vi "ADS Custom Personality FPGA FPGA.vi"() -> ()   [LabVIEW 2015]
uses:
  FPGA Function.ctl
  <vilib>/LabVIEW Targets/FPGA/cRIO/shared/nicrio_ModuleControls/nicrio_cRIO-9237_DataRatesRing.ctl
  <vilib>/LabVIEW Targets/FPGA/cRIO/shared/nicrio_ModuleControls/nicrio_cRIO-9237_ExcitationVoltageRing.ctl
  <vilib>/Platform/TimedLoop/XDataNode/timing_clust.ctl
  <vilib>/Platform/TimedLoop/XDataNode/nitl_modes.ctl
  <vilib>/Platform/TimedLoop/XDataNode/wakeup.ctl
  <vilib>/LabVIEW Targets/FPGA/cRIO/shared/nicrio_ModuleControls/nicrio_cRIO-9871_BaudRatePrescalerEnum.ctl
  <vilib>/LabVIEW Targets/FPGA/cRIO/shared/nicrio_ModuleControls/nicrio_cRIO-9871_XcvrModeEnum.ctl
  <vilib>/rvi/Emulation/niFpgaGetClockAttributes.vi
  <vilib>/rvi/Emulation/niFpgaSctlEmulationGetInTimedLoop.vi
  <vilib>/rvi/Emulation/niFpgaEmulationReportErrorSimple.vi
  <vilib>/rvi/Emulation/niFpgaCriticalErrorInLSC.vi
  <vilib>/rvi/eio/common/nirviEmuTemplateMethod_errors.vi
  <vilib>/rvi/eio/common/nirviEmuTemplatePropertySet_noerrors.vi
  <vilib>/rvi/Emulation/niFpgaProcessEmulError.vi
  <vilib>/rvi/DataTransferAndStorage/Container/Common/niFpgaContainerGetUniqueNameForEmu.vi
  <vilib>/rvi/DataTransferAndStorage/Container/Common/niFpgaContainerSetEmuInfo.vi
  <vilib>/rvi/eio/common/nirviEmuReportErrorAndStop.vi
  <vilib>/rvi/DataTransferAndStorage/Container/Common/niFpgaContainerExecOnDevCompGetState.vi
  <vilib>/rvi/Emulation/niFpgaEmulationIsFPGAContextNoSignature.vi
  <vilib>/rvi/errors/niFpgaSetErrorForExecOnDevCompSimple.vi
  <vilib>/rvi/FIFO/Fifo_Resource/nirvififoEmulationSetSize.vi
  <vilib>/rvi/FIFO/Fifo_Resource/nirviFifoEmulationQueueMgr.vi
  <instcachedir>/0/nirviFifoEmulationQueueMgr_E5CAEC123FF24DC58D834DCA3CDAA9B5.lvgen/nirviFifoEmulationQueueMgr_E5CAEC123FF24DC58D834DCA3CDAA9B5_001.vi
  <vilib>/rvi/FIFO/Fifo_Resource/nirvififoEmulationDetermineInputValidOut.vi
  <vilib>/rvi/FIFO/Fifo_Resource/nirvififoEmulationCreateLock.vi
  <vilib>/rvi/FIFO/Fifo_Resource/nirvififoEmulationObtainLock.vi
  <vilib>/rvi/FIFO/Fifo_Resource/nirvififoEmulationReleaseLock.vi
  <vilib>/rvi/occurrence/nirviWaitOnOccurrenceBase.vi
  <vilib>/rvi/errors/nirviReportUnexpectedCaseInternalError.vi
  <vilib>/rvi/errors/nirviReportUnexpectedCaseInternalError (U32).vi
  <vilib>/Utility/error.llb/Clear Errors.vi
  <vilib>/rvi/interface/RandomDataEmulation/niFpgaRandomDataHandleErrors.vi
  <vilib>/Platform/TimedLoop/XDataNode/XDataNode.xnode
  <vilib>/eio/EIONode/EIONode.xnode
  <vilib>/eio/EIOPropertyNode/EIOPropertyNode.xnode
  <vilib>/rvi/LocalResourceManager/LocalResourceManager.xnode
  <vilib>/rvi/DataTransferAndStorage/Container/XNode/niFpgaContainer.xnode
  <vilib>/rvi/FIFO/Fifo_Resource/niFpgaFifoEmulationRefIn.vi
  <vilib>/eio/EIOMethodNode/EIOMethodNode.xnode
  <vilib>/Platform/TimedLoop/XDataNode/XDNodeRunTimeDep.lvlib
  <vilib>/NI Veristand/FPGA/NI_VS FPGA Support.lvlib
  <userlib>/_NI VeriStand FPGA Support/NI VeriStand FPGA Clock Support/NI_VS FPGA Clock Support.lvlib
  <vilib>/rvi/eio/common/nirviEmuTemplatePropertyGet_errors.vi
  <vilib>/rvi/eio/common/nirviEmuTemplatePropertyGet_noerrors.vi
  <vilib>/rvi/eio/common/nirviEmuTemplatePropertySet_errors.vi
panel:
  out "Count 6":u32
  out "Count 5":u32
  out "Count 4":u32
  out "Count 3":u32
  out "Count 2":u32
  in  "Edge":enum8{"Either", "Rising Edge", "Falling Edge"}(ring)=enum."Rising Edge"
  in  "Reset":bool
  in  "Count Direction":enum16{"Count Down", "Count Up"}(ring)=enum."Count Up"
  out "Count":u32
  in  "Excitation Voltage":T1=2 items=["2.5 Volts", "3.3 Volts", "5.0 Volts", "10.0 Volts", "External Excitation"]
  in  "RecDelay":u32=550
  out "PosComm":fxp<+/-,24,16>[](array[numeric])=[68.78125, 0.0, 0.0, 0.0, 0.0, 0.0]
  in  "Baudrate":u8=4
  in  "SetBaudrate":bool
  out "Time":u32=1
  in  "Baud Rate Divider":u16=9
  in  "9237 Data Rate":T2=1 items=["50.000 kS/s (NI 9237)"=1, "25.000 kS/s (NI 9237)"=2, "16.667 kS/s (NI 9237)"=3, "12.500 kS/s (NI 9237)"=4, "10.000 kS/s (NI 9237)"=5, "8.333 kS/s (NI 9237)"=6, "7.143 kS/s (NI 9237)"=7, "6.250 kS/s (NI 9237)"=8, "5.556 kS/s (NI 9237)"=9, "5.000 kS/s (NI 9237)"=10, "4.545 kS/s (NI 9237)"=11, "4.167 kS/s (NI 9237)"=12, "3.846 kS/s (NI 9237)"=13, "3.571 kS/s (NI 9237)"=14, "3.333 kS/s (NI 9237)"=15, "3.125 kS/s (NI 9237)"=16, "2.941 kS/s (NI 9237)"=17, "2.778 kS/s (NI 9237)"=18, "2.632 kS/s (NI 9237)"=19, "2.500 kS/s (NI 9237)"=20, "2.381 kS/s (NI 9237)"=21, "2.273 kS/s (NI 9237)"=22, "2.174 kS/s (NI 9237)"=23, "2.083 kS/s (NI 9237)"=24, "2.000 kS/s (NI 9237)"=25, "1.923 kS/s (NI 9237)"=26, "1.852 kS/s (NI 9237)"=27, "1.786 kS/s (NI 9237)"=28, "1.724 kS/s (NI 9237)"=29, "1.667 kS/s (NI 9237)"=30, "1.613 kS/s (NI 9237)"=31]
  in  "NoB2Read":i32=48
  in  "ScaleDeg":fxp<+/-,25,16>=2.849609375
  out "ReadData":u8[](array[numeric])=[255, 255, 1, 4, 0, 196, 0, 54, 255, 255, 2, 4, 0, 0, 0, 249, 255, 255, 3, 4, 0, 0, 0, 248, 255, 255, 4, 4, 0, 0, 0, 247, 255, 255, 5, 4, 0, 0, 0, 246, 255, 255, 6, 4, 0, 0, 0, 245, 0, 0, 0, 0, 0, 0, 0, 0] format="%x"
  out "NoC":i32=49
  out "Number of Elements to Read Output":u32=26
  out "PresentPos":u64[](array[numeric])=[688, 0, 0, 210453397552]
  out "WriteData":u8[](array[numeric])=[255, 255, 254, 21, 146, 0, 2, 1, 36, 2, 2, 36, 2, 3, 36, 2, 4, 36, 2, 5, 36, 2, 6, 36, 97, 0, 0, 0, 0, 0]
  out "error out":errorcluster
  in  "SerialFunction":T3=enum."Read"
  in  "PosVal":fxp<+/-,24,16>
  in  "EOS Enabled":bool
  in  "EOS":u8
  out "Timed Out Read":bool
  out "EOS?":bool
  out "Timed Out Write":bool
  in  "_PWM Pulses 0-7":u64[](array[numeric])=[4294967395000, 100000, 100000, 100000, 100000, 100000, 100000, 100000]
  in  "Generate IRQ":bool=TRUE
  in  "Use External Timing":bool
  in  "Write to  RTSI":bool=TRUE
  in  "Loop Rate (usec)":u32=10000
  in  "Start":bool
  # "PWM"
  # "Configuration"
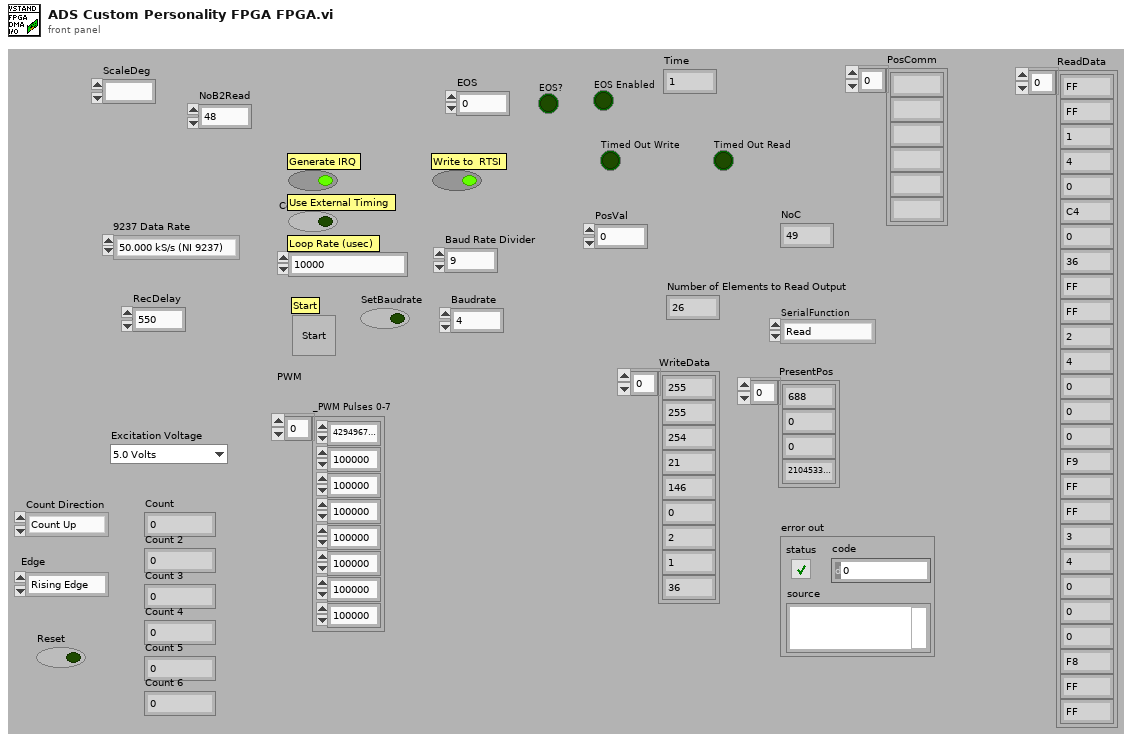
[diagram p1: front panel]
types:
  T1 = typedef "nicrio_cRIO-9237_ExcitationVoltageRing.ctl" = u8
  T2 = typedef "nicrio_cRIO-9237_DataRatesRing.ctl" = u8
  T3 = typedef "FPGA Function.ctl" = enum16{"Do Nothing", "Write", "Read"}
  T4 = typedef "XDNodeRunTimeDep.lvlib/timing_clust.ctl" = cluster{"Expected End [f-1]":u64, "Actual End [f-1]":u64, "Finished Late? [f-1]":bool, "Expected End [i-1]":u64, "Actual End [i-1]":u64, "Finished Late? [i-1]":bool, "Expected Start [i]":u64, "Actual Start [i]":u64, "Expected Start [f]":u64, "Actual Start [f]":u64, "Source Name":string, "Structure Name":string, "Period":i64, "Deadline":i64, "Offset":i64, "Start":i64, "Priority":i32, "Timeout":i32, "Mode":T5, "Wakeup Reason":T6, "Error":errorcluster, "Source Type":string, "Secondary Source Type":string, "Global End Time":u64, "Global Start Time":u64, "Frame Duration":u64, "Iteration Duration":u64, "Assigned CPU":i32, "I/O Scan Engine Mode":u32}
  T5 = typedef "XDNodeRunTimeDep.lvlib/nitl_modes.ctl" = enum32{"No Change", "Process missed periods, maintain original phase", "Discard missed periods, maintain original phase", "Process missed periods, ignore original phase", "Discard missed periods, ignore original phase"}
  T6 = typedef "XDNodeRunTimeDep.lvlib/wakeup.ctl" = enum32{"Normal", "Aborted", "Asynchronous wakeup", "Timing source error", "Timed loop error", "Timeout"}
  T7 = cluster{"9235/9236/9237 AI0":refnum<k21>, "9235/9236/9237 AI1":refnum<k21>, "9235/9236/9237 AI2":refnum<k21>, "9235/9236/9237 AI3":refnum<k21>}
  T8 = cluster{"9215 AI0":refnum<k21>, "9215 AI1":refnum<k21>, "9215 AI2":refnum<k21>, "9215 AI3":refnum<k21>}
  T9 = typedef "nicrio_cRIO-9871_XcvrModeEnum.ctl" = enum8{"4 Wire", "2 Wire DTR Controlled with Echo", "2 Wire DTR Controlled", "2 Wire Auto"}
  T10 = typedef "nicrio_cRIO-9871_BaudRatePrescalerEnum.ctl" = enum8{"1", "4"}
  T11 = cluster{"DO0":refnum<k21>, "DO1":refnum<k21>, "DO2":refnum<k21>, "DO3":refnum<k21>}
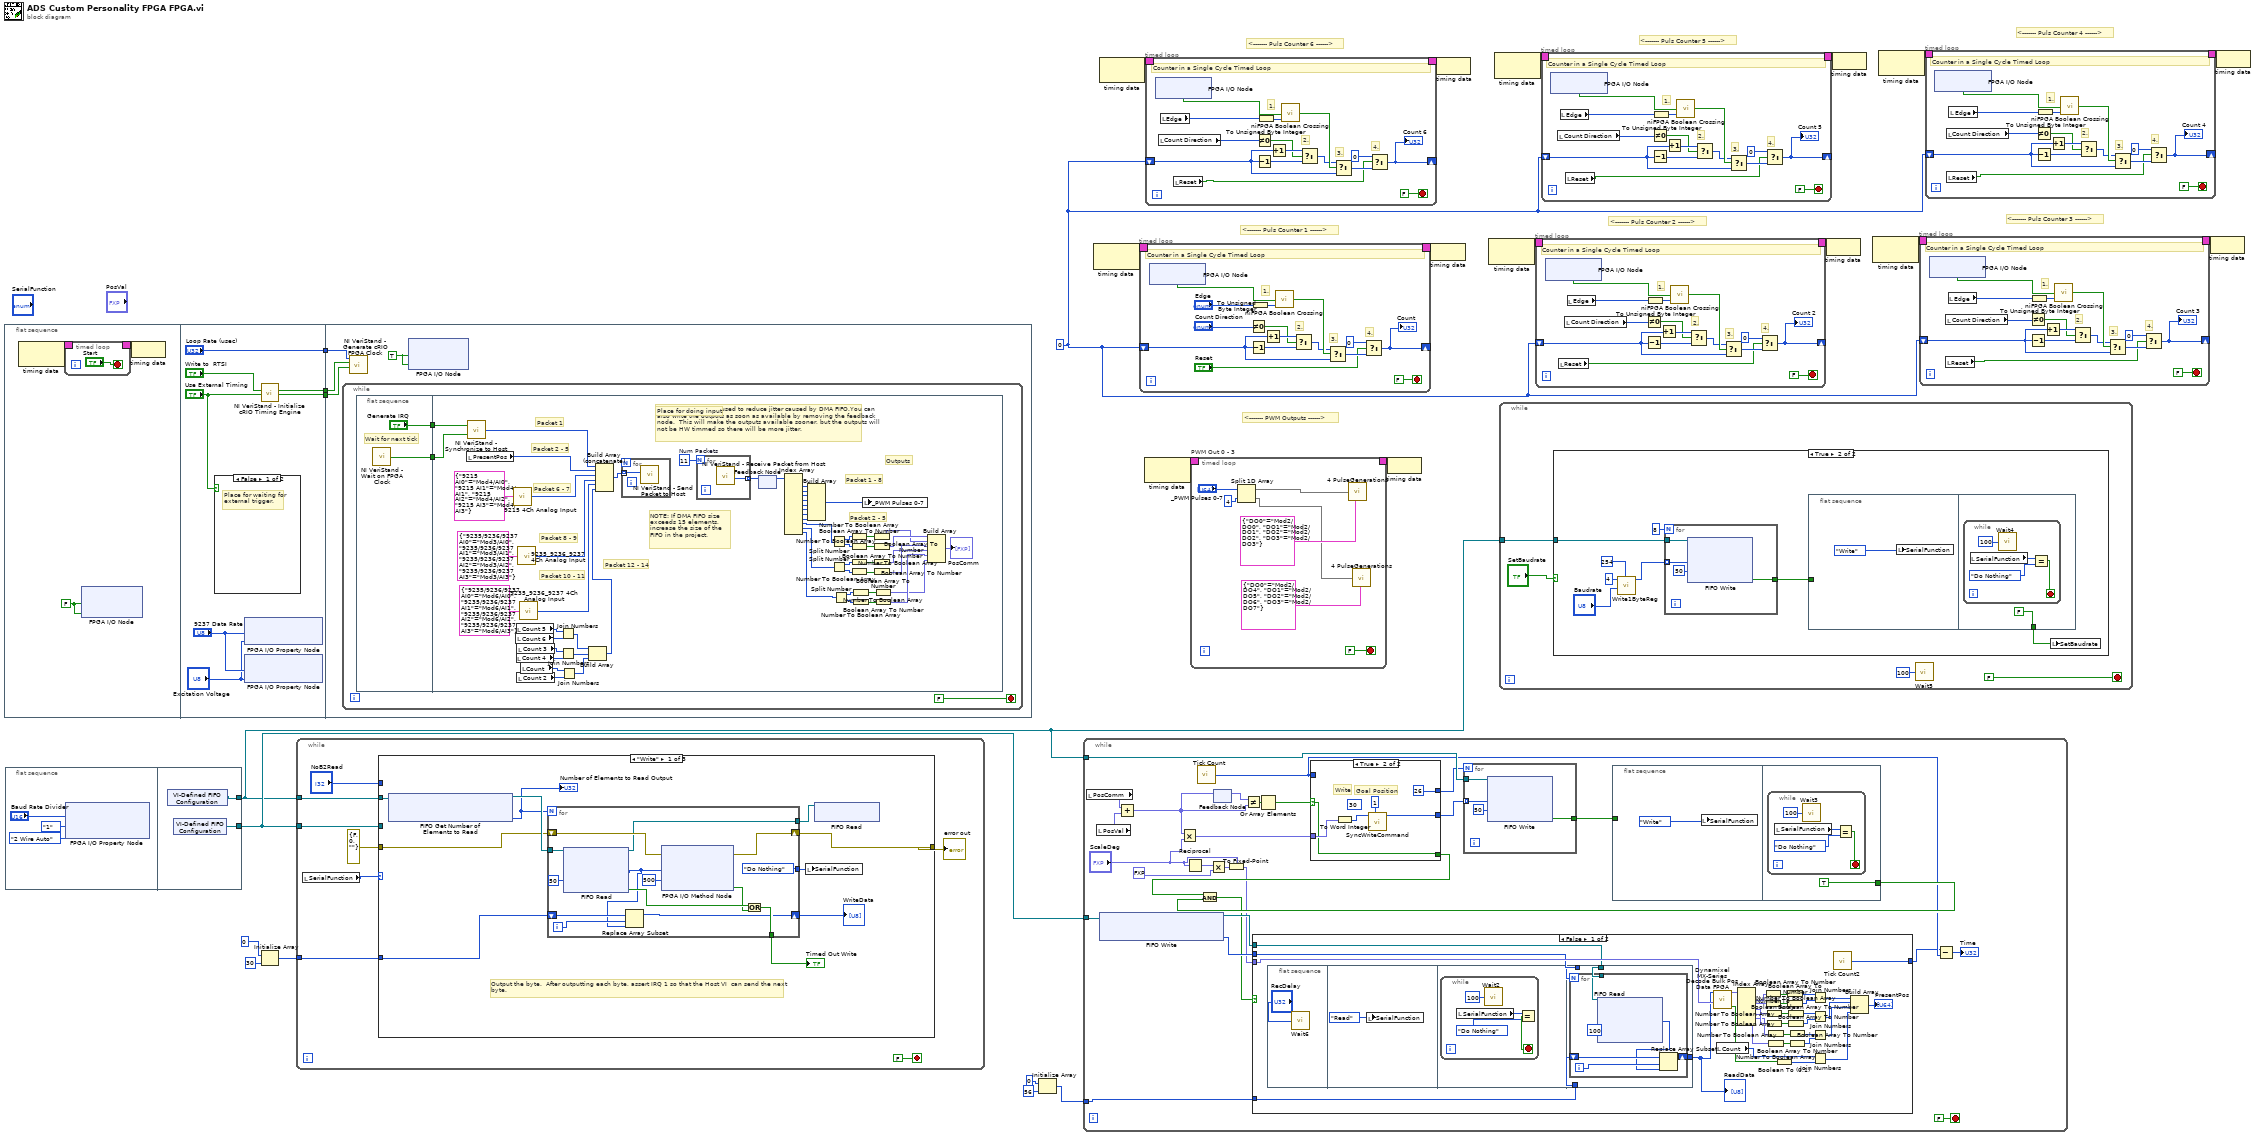
[diagram p0: block diagram]
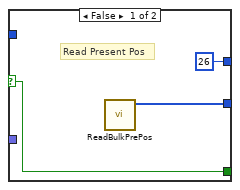
[diagram p4: hidden frame]
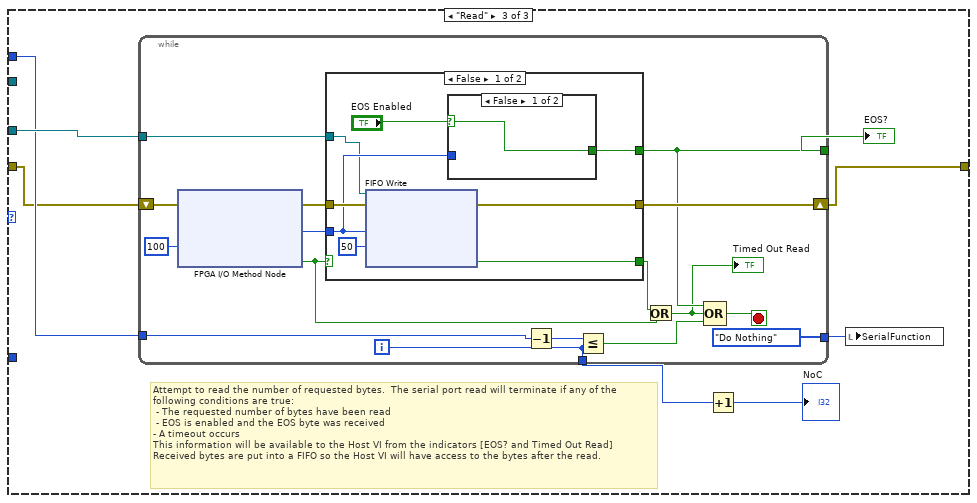
[diagram p6: hidden frame]
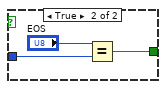
[diagram p7: hidden frame]
diagram:
  w1 = u32 0
  # "<------- Puls Counter 5 ------>"
  # "<------- Puls Counter 4 ------>"
  # "<------- Puls Counter 3 ------>"
  # "<------- Puls Counter 2 ------>"
  # "<------- Puls Counter 6 ------>"
  # "<------- Puls Counter 1 ------>"
  # "<------- PWM Outputs ------>"
  n1 = flat-sequence {
    tunnel: [w38] -> w26
    tunnel: ["Loop Rate (usec)"] -> w25
    tunnel: [w37] -> w22
    tunnel: w26 -> [w45]
    tunnel: w25 -> [w44]
    tunnel: w22 -> [w43]
    frame #0 {
      w27 = FALSE
      n2 = node-c288() -> (w29:T4)  [unwired: 1 out]
      n3 = timed-loop {
        timing: w29 -> [_]
        timing-out: [_] -> w28
        stop <- "Start" stop-if-true
      }
      n4 = xnode "FPGA I/O Node"("Mod3/Start"=w27, "Mod6/Start"=w27) -> ()  [unwired: 2 in, 2 out]
      n5 = node-c288(w28) -> ()
    }
    frame #1 {
      n6 = case shown="False" "Use External Timing" {
        frame False {
          # "Place for waiting for external trigger."
        }
        frame True {
          # "Do not wait on trigger when externally timed."
        }
      }
      n7 = xnode "FPGA I/O Property Node"("Data Rate"="9237 Data Rate", "Excitation Voltage"="Excitation Voltage") -> ()  [unwired: 1 in, 1 out]
      n8 = xnode "FPGA I/O Property Node"("Data Rate"="9237 Data Rate", "Excitation Voltage"="Excitation Voltage") -> ()  [unwired: 1 in, 1 out]
      n9 = call <userlib>:"NI VeriStand - Initialize cRIO Timing Engine.vi"("Use External Timing In"="Use External Timing", "Write to  RTSI In"="Write to  RTSI") -> ("Use External Timing Out"=w38:bool, "Write to  RTSI Out"=w37:bool)  [unwired: 8 in]
    }
    frame #2 {
      w42 = TRUE
      n10 = while {
        stop <- FALSE stop-if-true
        n11 = flat-sequence {
          tunnel: ["Generate IRQ"] -> w47
          tunnel: [w49] -> w46
          tunnel: w47 -> [w105]
          tunnel: w46 -> [w104]
          frame #0 {
            # "Wait for next tick"
            n12 = call <userlib>:"NI VeriStand - Wait on FPGA Clock.vi"() -> ("Clock Ticked"=w49:bool)
          }
          frame #1 {
            w103 = 11  # Num Packets
            # "Packet 12 - 14"
            # "Packet 10 - 11"
            # "Packet 1"
            # "Packet 6 - 7"
            # "Outputs"
            # "Packet 2 - 5"
            # "Packet 8 - 9"
            # "Packet 2 - 5"
            # "Packet 1 - 8"
            # "NOTE: If DMA FIFO size exceeds 15 elements, increase the size of the FIFO in the project."
            # "Feedback nodes are used to reduce jitter caused by DMA FIFO.You can also write the outputs as soon as available by removing the feedback node.  This will make the outputs available sooner, but the outputs will not be HW timmed so there will be more jitter."
            # "Place for doing input"
            n13 = local read "PresentPos"() -> (w85:u64[])
            n14 = call <userlib>:"NI VeriStand - Synchronize to Host.vi"("Clock Ticked"=w104, "Generate IRQ"=w105) -> ("Is Late?"=w98:u64)
            n15 = call <userlib>:"9215 4Ch Analog Input.vi"("9215 I/O"=T8 {"9215 AI0"="Mod4/AI0", "9215 AI1"="Mod4/AI1", "9215 AI2"="Mod4/AI2", "9215 AI3"="Mod4/AI3"}) -> ("Packets"=w87:u64[])
            n16 = local read "Count 6"() -> (w59:u32)
            n17 = local read "Count 5"() -> (w60:u32)
            n18 = local read "Count 4"() -> (w58:u32)
            n19 = local read "Count 3"() -> (w57:u32)
            n20 = local read "Count 2"() -> (w55:u32)
            n21 = call <userlib>:"9235_9236_9237 4Ch Analog Input.vi"("9235/9236/9237 I/O"=T7 {"9235/9236/9237 AI0"="Mod3/AI0", "9235/9236/9237 AI1"="Mod3/AI1", "9235/9236/9237 AI2"="Mod3/AI2", "9235/9236/9237 AI3"="Mod3/AI3"}) -> ("Packets"=w86:u64[])
            n22 = call <userlib>:"9235_9236_9237 4Ch Analog Input.vi"("9235/9236/9237 I/O"=T7 {"9235/9236/9237 AI0"="Mod6/AI0", "9235/9236/9237 AI1"="Mod6/AI1", "9235/9236/9237 AI2"="Mod6/AI2", "9235/9236/9237 AI3"="Mod6/AI3"}) -> ("Packets"=w61:u64[])
            n23 = local read "Count"() -> (w56:u32)
            n24 = Join Numbers(hi=w60, lo=w59) -> ((hi.lo)=w54:u64)
            n25 = Join Numbers(hi=w57, lo=w58) -> ((hi.lo)=w53:u64)
            n26 = Join Numbers(hi=w56, lo=w55) -> ((hi.lo)=w52:u64)
            n27 = Build Array(w54, w53, w52) -> (w51:u64[])
            n28 = Build Array (concatenate)(w98, w85, w87, w86, w61, w51) -> (w97:u64[])
            n29 = for {
              tunnel: w97 -> [w106] mode=indexing
              n30 = call <vilib>:"NI VeriStand - Send Packet to Host.vi"("Element"=w106) -> ()  [unwired: 2 in, 9 out]
            }
            n31 = for {
              N: w103 -> [_]
              tunnel: [w107] -> w94 mode=indexing
              n32 = call <vilib>:"NI VeriStand - Receive Packet from Host.vi"() -> ("Element"=w107:u64)  [unwired: 2 in, 9 out]
            }
            n33 = feedback-in #1(w94) -> ()
            n34 = feedback #1() -> (w95:u64[])  [unwired: 1 in]
            n35 = Index Array(array=w95) -> (element #1=w91:u64, element #2=w102:u64, element #3=w101:u64, element #4=w100:u64, element #5=w99:u64, element #6=w92:u64, element #7=w90:u64, element #8=w89:u64, element #9=w80:u64, element #10=w71:u64, element #11=w70:u64)  [unwired: 11 in]
            n36 = Build Array(w91, w102, w101, w100, w99, w92, w90, w89) -> (w96:u64[])
            n37 = Split Number(x=w80) -> (hi(x)=w82:u32, lo(x)=w81:u32)
            n38 = Split Number(x=w71) -> (hi(x)=w78:u32, lo(x)=w79:u32)
            n39 = Split Number(x=w70) -> (hi(x)=w73:u32, lo(x)=w72:u32)
            n40 = Number To Boolean Array(number=w82) -> (Boolean array=w83:bool[])
            n41 = Number To Boolean Array(number=w81) -> (Boolean array=w84:bool[])
            n42 = Number To Boolean Array(number=w78) -> (Boolean array=w77:bool[])
            n43 = Number To Boolean Array(number=w79) -> (Boolean array=w76:bool[])
            n44 = Number To Boolean Array(number=w73) -> (Boolean array=w74:bool[])
            n45 = Number To Boolean Array(number=w72) -> (Boolean array=w75:bool[])
            n46 = local write "_PWM Pulses 0-7"(w96) -> ()
            n47 = Boolean Array To Number(Boolean array=w83) -> (number=w68:fxp<+/-,24,16>)
            n48 = Boolean Array To Number(Boolean array=w84) -> (number=w69:fxp<+/-,24,16>)
            n49 = Boolean Array To Number(Boolean array=w77) -> (number=w66:fxp<+/-,24,16>)
            n50 = Boolean Array To Number(Boolean array=w76) -> (number=w67:fxp<+/-,24,16>)
            n51 = Boolean Array To Number(Boolean array=w74) -> (number=w64:fxp<+/-,24,16>)
            n52 = Boolean Array To Number(Boolean array=w75) -> (number=w65:fxp<+/-,24,16>)
            n53 = Build Array(w69, w68, w67, w66, w65, w64) -> (→"PosComm":fxp<+/-,24,16>[])
          }
        }
      }
      n54 = call <userlib>:"NI VeriStand - Generate cRIO FPGA Clock.vi"("Use External Timing"=w45, "Write to  RTSI"=w43, "Loop Rate (usec)"=w44) -> ()  [unwired: 9 in]
      n55 = xnode "FPGA I/O Node"("Mod3/Start"=w42, "Mod6/Start"=w42) -> ()  [unwired: 2 in, 2 out]
    }
  }
  n56 = flat-sequence {
    tunnel: [w112] -> w14
    tunnel: [w111] -> w21
    frame #0 {
      n57 = xnode "FPGA I/O Property Node"("Baud Rate Divider"="Baud Rate Divider", "Baud Rate Prescaler"=nicrio_cRIO-9871_BaudRatePrescalerEnum."1", "Transceiver Mode"=nicrio_cRIO-9871_XcvrModeEnum."2 Wire Auto") -> ()  [unwired: 1 in, 1 out]
    }
    frame #1 {
      n58 = xnode "VI-Defined FIFO Configuration"() -> ("FIFO Out"=w112:refnum<k21>)
      n59 = xnode "VI-Defined FIFO Configuration"() -> ("FIFO Out"=w111:refnum<k21>)
    }
  }
  n60 = Initialize Array(u8 0 ("Element"), 30 ("dimension size")) -> (w16:u8[])
  n61 = while {
    tunnel: w21 -> [w120]
    tunnel: w14 -> [w117]
    tunnel: w16 -> [w113]
    stop <- FALSE stop-if-true
    n62 = local read "SerialFunction"() -> (w119:T3)
    n63 = case shown="\"Write\"" w119 {
      tunnel: [w130 w145 w153] -> w115
      tunnel: w120 -> [_ _ w151]
      tunnel: "NoB2Read" -> [_ _ w150]
      tunnel: w117 -> [w129 _ _]
      tunnel: errorcluster {"status"=FALSE, "code"=0, "source"=""} ("error out") -> [w126 w145 w149]
      tunnel: w113 -> [w122 _ _]
      frame "Write" {
        # "Output the byte.  After outputting each byte, assert IRQ 1 so that the Host VI  can send the next \nbyte."
        n64 = xnode ("FIFO Get Number of Elements to Read")("FIFO In"=w129) -> ("Number of Elements to Read"=w121:u32, "FIFO Out"=w128:refnum<k21>)
        "Number of Elements to Read Output" <- w121
        n65 = for {
          N: w121 -> [_]
          tunnel: w128 -> [w142]
          tunnel: [w140] -> w127
          shift-right: [w144] -> w130
          shift-left: w126 -> [w137]
          tunnel: [w136] -> w125
          shift-right: [w134] -> w124
          shift-left: w122 -> [w135]
          tunnel: [FPGA_Function."Do Nothing" ("SerialFunction")] -> w123
          i -> [w133]
          n66 = xnode ("FIFO Read")("Timeout"=50, "FIFO In"=w142) -> ("Element"=w132:u8, "Timed Out?"=w139:bool, "FIFO Out"=w136:refnum<k21>)
          n67 = Replace Array Subset(array=w135, new element=w132, index=w133) -> (w134:u8[])
          n68 = xnode "FPGA I/O Method Node"("error in"=w137, "Data"=w132, "Timeout (ms)"=500) -> ("error out"=w144:errorcluster, "Timed Out"=w138:bool)  [unwired: 1 in, 1 out]
          n69 = Or(x=w139, y=w138) -> (x .or. y?=w140:bool)
        }
        "Timed Out Write" <- w127
        "WriteData" <- w124
        n70 = local write "SerialFunction"(w123) -> ()
        n71 = xnode ("FIFO Read")("FIFO In"=w125) -> ()  [unwired: 1 out]
      }
      frame "Do Nothing", Default {
        # "Do Nothing"
      }
      frame "Read" {
        # "Attempt to read the number of requested bytes.  The serial port read will terminate if any of the \nfollowing conditions are true:\n - The requested number of bytes have been read\n - EOS is enabled and the EOS byte was received\n- A timeout occurs\nThis information will be available to the Host VI from the indicators [EOS? and Timed Out Read]\nReceived bytes are put into a FIFO so the Host VI will have access to the bytes after the read."
        n72 = while {
          shift-right: [w169] -> w153
          shift-left: w149 -> [w167]
          tunnel: [w162] -> w152
          tunnel: w151 -> [w154]
          tunnel: w150 -> [w159]
          tunnel: [FPGA_Function."Do Nothing" ("SerialFunction")] -> w148
          tunnel: [w157] -> w147
          i -> [w157]
          stop <- w166 stop-if-true
          n73 = xnode "FPGA I/O Method Node"("error in"=w167, "Timeout (ms)"=100) -> ("error out"=w168:errorcluster, "Data"=w156:u8, "Timed Out"=w155:bool)  [unwired: 1 in, 1 out]
          n74 = case shown="False" w155 {
            selector: w155 -> [_ w182]
            tunnel: [w177 w182] -> w163
            tunnel: w156 -> [w173 _]
            tunnel: [w175 w183] -> w169
            tunnel: w168 -> [w174 w183]
            tunnel: [w171 _] -> w162
            tunnel: w154 -> [w170 _]
            frame False {
              n75 = xnode ("FIFO Write")("Element"=w173, "Timeout"=50, "error in (no error)"=w174, "FIFO In"=w170) -> ("Timed Out?"=w177:bool, "error out"=w175:errorcluster)  [unwired: 1 out]
              n76 = case shown="False" "EOS Enabled" {
                selector: "EOS Enabled" -> [w178 _]
                tunnel: [w178 w180] -> w171
                tunnel: w173 -> [_ w179]
                frame False {
                }
                frame True {
                  n77 = Equal?(x="EOS", y=w179) -> (x = y?=w180:bool)
                }
              }
            }
            frame True {
            }
          }
          n78 = Decrement(x=w159) -> (x-1=w165:i32)
          n79 = Less Or Equal?(x=w165, y=w157) -> (x <= y?=w164:bool)
          n80 = Or(x=w163, y=w155) -> (x .or. y?=w161:bool)
          "Timed Out Read" <- w161
          n81 = Compound Arithmetic op=OR(w162, w161, w164) -> (w166:bool)
        }
        "EOS?" <- w152
        n82 = Increment(x=w147) -> (x+1=→"NoC":i32)
        n83 = local write "SerialFunction"(w148) -> ()
      }
    }
    "error out" <- w115
  }
  n84 = Initialize Array(u8 0 ("Element"), 56 ("dimension size")) -> (w15:u8[])
  n85 = while {
    tunnel: w14 -> [w204]
    tunnel: w21 -> [w196]
    tunnel: w15 -> [w199]
    stop <- FALSE stop-if-true
    n86 = local read "PosComm"() -> (w203:fxp<+/-,24,16>[])
    n87 = local read "PosVal"() -> (w201:fxp<+/-,24,16>)
    n88 = xnode ("FIFO Write")("FIFO In"=w196) -> ("Number of Elements to Read"=w194:u32, "FIFO Out"=w195:refnum<k21>)  [unwired: 1 in, 1 out]
    n89 = Add(x=w203, y=w201) -> (x+y=w198:fxp<+/-,25,17>[])
    n90 = Multiply(x=w198, y="ScaleDeg") -> (x*y=w197:fxp<+/-,50,33>[])
    n91 = Reciprocal(x="ScaleDeg") -> (1/x=w187:fxp<+/-,27,11>)
    n92 = call "Tick Count"() -> ("Tick Count(mSec)"=w192:u32)
    n93 = Multiply(x=w187, y=fxp<+,25,16> 10.0) -> (x*y=w186:fxp<+/-,51,26>)
    n94 = feedback #2() -> (w209:fxp<+/-,25,17>[])  [unwired: 1 in]
    n95 = feedback-in #2(w198) -> ()
    n96 = To Fixed-Point(fixed-point type="ScaleDeg", number=w186) -> (fixed-point=w193:fxp<+/-,25,16>)
    n97 = Not Equal?(x=w209, y=w198) -> (x != y?=w208:bool[])
    n98 = Or Array Elements(Boolean array=w208) -> (logical OR=w185:bool)
    n99 = case shown="True" w185 {
      selector: w185 -> [w272 w276]
      tunnel: w197 -> [_ w277]
      tunnel: [w271 w273] -> w206
      tunnel: [w272 w276] -> w205
      tunnel: [26 26 ("length")] -> w202
      tunnel: w192 -> [_ _]
      frame False {
        # "Read Present Pos"
        n100 = call "ReadBulkPrePos.vi"() -> ("Data"=w271:u8[])  [unwired: 10 in, 1 out]
      }
      frame True {
        (unwired) u8 30 ("RegAddr")
        # "Write"
        # "Goal Position"
        n101 = To Word Integer(number=w277) -> (16bit integer=w275:i16[])
        n102 = call "SyncWriteCommand.vi"("MxID"=u8 1, "PosParm"=w275) -> ("Data"=w273:u8[])  [unwired: 8 in, 1 out]
      }
    }
    n103 = And(x=w205, y=w200) -> (x .and. y?=w184:bool)
    n104 = case shown="False" w184 {
      tunnel: w195 -> [w245 _]
      tunnel: w199 -> [w246 _]
      tunnel: w194 -> [w239 _]
      tunnel: w193 -> [w248 _]
      tunnel: [w247 _] -> w191
      frame False {
        n105 = flat-sequence {
          tunnel: w246 -> [w259]
          tunnel: w245 -> [w258]
          tunnel: w239 -> [w257]
          tunnel: [w256] -> w244
          frame #0 {
            n106 = call "Wait6"("Count(uSec)"="RecDelay") -> ()  [unwired: 1 out]
          }
          frame #1 {
            n107 = local write "SerialFunction"(FPGA_Function."Read" ("Op Control")) -> ()
          }
          frame #2 {
            n108 = while {
              stop <- w254 stop-if-true
              n109 = local read "SerialFunction"() -> (w253:T3)
              n110 = call "Wait2"("Count(uSec)"=u32 100) -> ()  [unwired: 1 out]
              n111 = Equal?(x=w253, y=FPGA_Function."Do Nothing" ("SerialFunction")) -> (x = y?=w254:bool)
            }
          }
          frame #3 {
            n112 = for {
              N: w257 -> [_]
              shift-right: [w264] -> w256
              shift-left: w259 -> [w263]
              tunnel: w258 -> [w262]
              i -> [w265]
              n113 = xnode ("FIFO Read")("Timeout"=100, "FIFO In"=w262) -> ("Element"=w260:u8)  [unwired: 2 out]
              n114 = Replace Array Subset(array=w263, new element=w260, index=w265) -> (w264:u8[])
            }
          }
        }
        n115 = call "Dynamixel MX-Series Decode Bulk Pos Data FPGA.vi"("ScaleOutput"=w248, "RecData"=w244) -> ("CError"=w236:bool, "Position"=w242:fxp<+/-,24,16>[])  [unwired: 7 in, 1 out]
        n116 = local read "Count"() -> (w237:u32)
        n117 = Index Array(array=w242) -> (element #1=w229:fxp<+/-,24,16>, element #2=w230:fxp<+/-,24,16>, element #3=w220:fxp<+/-,24,16>, element #4=w219:fxp<+/-,24,16>, element #5=w218:fxp<+/-,24,16>, element #6=w217:fxp<+/-,24,16>)  [unwired: 6 in]
        n118 = Number To Boolean Array(number=w229) -> (Boolean array=w234:bool[])
        n119 = Number To Boolean Array(number=w230) -> (Boolean array=w233:bool[])
        n120 = Number To Boolean Array(number=w220) -> (Boolean array=w227:bool[])
        n121 = Number To Boolean Array(number=w219) -> (Boolean array=w228:bool[])
        n122 = Number To Boolean Array(number=w218) -> (Boolean array=w226:bool[])
        n123 = Number To Boolean Array(number=w217) -> (Boolean array=w225:bool[])
        n124 = Boolean To (0,1)(Boolean=w236) -> (0, 1=w235:i16)
        n125 = Boolean Array To Number(Boolean array=w234) -> (number=w231:u32)
        n126 = Boolean Array To Number(Boolean array=w233) -> (number=w232:u32)
        n127 = Boolean Array To Number(Boolean array=w227) -> (number=w223:u32)
        n128 = Boolean Array To Number(Boolean array=w228) -> (number=w222:u32)
        n129 = Boolean Array To Number(Boolean array=w226) -> (number=w221:u32)
        n130 = Boolean Array To Number(Boolean array=w225) -> (number=w224:u32)
        n131 = Join Numbers(hi=w231, lo=w232) -> ((hi.lo)=w243:u64)
        n132 = Join Numbers(hi=w223, lo=w222) -> ((hi.lo)=w241:u64)
        n133 = Join Numbers(hi=w221, lo=w224) -> ((hi.lo)=w240:u64)
        n134 = Join Numbers(hi=w237, lo=w235) -> ((hi.lo)=w238:u64)
        n135 = call "Tick Count2"() -> ("Tick Count(mSec)"=w247:u32)
        n136 = Build Array(w243, w241, w240, w238) -> (→"PresentPos":u64[])
        "ReadData" <- w244
      }
      frame True {
      }
    }
    n137 = for {
      N: w202 -> [_]
      tunnel: w204 -> [w269]
      tunnel: w206 -> [w268] mode=indexing
      tunnel: [w267] -> w207
      n138 = xnode ("FIFO Write")("Element"=w268, "Timeout"=50, "FIFO In"=w269) -> ("Timed Out?"=w267:bool)  [unwired: 1 out]
    }
    n139 = flat-sequence {
      tunnel: w207 -> [_]
      tunnel: [TRUE] -> w200
      frame #0 {
        n140 = local write "SerialFunction"(FPGA_Function."Write" ("Op Control")) -> ()
      }
      frame #1 {
        n141 = while {
          stop <- w215 stop-if-true
          n142 = local read "SerialFunction"() -> (w214:T3)
          n143 = call "Wait3"("Count(uSec)"=u32 100) -> ()  [unwired: 1 out]
          n144 = Equal?(x=w214, y=FPGA_Function."Do Nothing" ("SerialFunction")) -> (x = y?=w215:bool)
        }
      }
    }
    n145 = Subtract(x=w191, y=w192) -> (x-y=→"Time":u32)
  }
  n146 = node-c288() -> (w13:T4)  [unwired: 1 in]
  n147 = node-c288() -> (w7:T4)  [unwired: 1 in]
  n148 = timed-loop "Timed Loop" {
    timing: w13 -> [_]
    timing-out: [_] -> w12
    shift-right: [w291] -> _
    shift-left: w1 -> [w287]
    stop <- FALSE stop-if-true
    # "3."
    # "4."
    # "2."
    # "1."
    # "Counter in a Single Cycle Timed Loop"
    n149 = xnode "FPGA I/O Node"() -> ("Mod5/DI0"=w280:bool)  [unwired: 1 in, 1 out]
    n150 = Not Equal To 0?(x="Count Direction") -> (x != 0?=w284:bool)
    n151 = Decrement(x=w287) -> (x-1=w288:u32)
    n152 = To Unsigned Byte Integer(number="Edge") -> (unsigned 8bit integer=w281:u8)
    n153 = Increment(x=w287) -> (x+1=w286:u32)
    n154 = call <vilib>:"niFPGA Boolean Crossing.vi"("input"=w280, "direction"=w281) -> ("crossing"=w293:bool)  [unwired: 7 in]
    n155 = Select(t=w286, s=w284, f=w288) -> (s? t:f=w283:u32)
    n156 = Select(t=w283, s=w293, f=w287) -> (s? t:f=w292:u32)
    n157 = Select(t=u32 0, s="Reset", f=w292) -> (s? t:f=w291:u32)
    "Count" <- w291
  }
  n158 = node-c288() -> (w24:T4)  [unwired: 1 out]
  n159 = timed-loop "Timed Loop" {
    timing: w7 -> [_]
    timing-out: [_] -> w6
    shift-right: [w308] -> _
    shift-left: w1 -> [w305]
    stop <- FALSE stop-if-true
    # "3."
    # "4."
    # "2."
    # "1."
    # "Counter in a Single Cycle Timed Loop"
    n160 = xnode "FPGA I/O Node"() -> ("Mod5/DI5"=w300:bool)  [unwired: 1 in, 1 out]
    n161 = local read "Count Direction"() -> (w297:enum16{"Count Down", "Count Up"})
    n162 = local read "Edge"() -> (w298:enum8{"Either", "Rising Edge", "Falling Edge"})
    n163 = local read "Reset"() -> (w296:bool)
    n164 = Not Equal To 0?(x=w297) -> (x != 0?=w303:bool)
    n165 = Decrement(x=w305) -> (x-1=w306:u32)
    n166 = To Unsigned Byte Integer(number=w298) -> (unsigned 8bit integer=w301:u8)
    n167 = Increment(x=w305) -> (x+1=w304:u32)
    n168 = call <vilib>:"niFPGA Boolean Crossing.vi"("input"=w300, "direction"=w301) -> ("crossing"=w310:bool)  [unwired: 7 in]
    n169 = Select(t=w304, s=w303, f=w306) -> (s? t:f=w302:u32)
    n170 = Select(t=w302, s=w310, f=w305) -> (s? t:f=w309:u32)
    n171 = Select(t=u32 0, s=w296, f=w309) -> (s? t:f=w308:u32)
    "Count 6" <- w308
  }
  n172 = timed-loop "PWM Out 0 - 3" {
    timing: w24 -> [_]
    timing-out: [_] -> w23
    stop <- FALSE stop-if-true
    n173 = Split 1D Array(array="_PWM Pulses 0-7", index=4 ("length")) -> (first subarray=w314:u64[], second subarray=w313:u64[])
    n174 = call <userlib>:"4 PulseGenerations.vi"("PulseGen Packets"=w314, "4 PulseGen Chs"=T11 {"DO0"="Mod2/DO0", "DO1"="Mod2/DO1", "DO2"="Mod2/DO2", "DO3"="Mod2/DO3"}) -> ()  [unwired: 8 in]
    n175 = call <userlib>:"4 PulseGenerations.vi"("PulseGen Packets"=w313, "4 PulseGen Chs"=T11 {"DO0"="Mod2/DO4", "DO1"="Mod2/DO5", "DO2"="Mod2/DO6", "DO3"="Mod2/DO7"}) -> ()  [unwired: 8 in]
  }
  n176 = node-c288(w23) -> ()
  n177 = node-c288(w12) -> ()
  n178 = node-c288(w6) -> ()
  n179 = node-c288() -> (w11:T4)  [unwired: 1 in]
  n180 = node-c288() -> (w5:T4)  [unwired: 1 in]
  n181 = while {
    tunnel: w14 -> [w323]
    stop <- FALSE stop-if-true
    n182 = case shown="True" "SetBaudrate" {
      tunnel: w323 -> [_ w328]
      frame False {
      }
      frame True {
        n183 = call "Write1ByteReg.vi"("MxID"=u8 254, "Param"="Baudrate", "RegAddr"=u8 4) -> ("Data"=w329:u8[])  [unwired: 7 in, 1 out]
        n184 = for {
          N: 8 -> [_]
          tunnel: w328 -> [w343]
          tunnel: w329 -> [w342] mode=indexing
          tunnel: [w341] -> w327
          n185 = xnode ("FIFO Write")("Element"=w342, "Timeout"=50, "FIFO In"=w343) -> ("Timed Out?"=w341:bool)  [unwired: 1 out]
        }
        n186 = flat-sequence {
          tunnel: w327 -> [_]
          tunnel: [FALSE] -> w326
          frame #0 {
            n187 = local write "SerialFunction"(FPGA_Function."Write" ("Op Control")) -> ()
          }
          frame #1 {
            n188 = while {
              stop <- w338 stop-if-true
              n189 = local read "SerialFunction"() -> (w337:T3)
              n190 = call "Wait4"("Count(uSec)"=u32 100) -> ()  [unwired: 1 out]
              n191 = Equal?(x=w337, y=FPGA_Function."Do Nothing" ("SerialFunction")) -> (x = y?=w338:bool)
            }
          }
        }
        n192 = local write "SetBaudrate"(w326) -> ()
      }
    }
    n193 = call "Wait5"("Count(mSec)"=u32 100) -> ()  [unwired: 1 out]
  }
  n194 = timed-loop "Timed Loop" {
    timing: w11 -> [_]
    timing-out: [_] -> w10
    shift-right: [w356] -> _
    shift-left: w1 -> [w353]
    stop <- FALSE stop-if-true
    # "3."
    # "4."
    # "2."
    # "1."
    # "Counter in a Single Cycle Timed Loop"
    n195 = xnode "FPGA I/O Node"() -> ("Mod5/DI1"=w348:bool)  [unwired: 1 in, 1 out]
    n196 = local read "Reset"() -> (w344:bool)
    n197 = local read "Count Direction"() -> (w345:enum16{"Count Down", "Count Up"})
    n198 = local read "Edge"() -> (w346:enum8{"Either", "Rising Edge", "Falling Edge"})
    n199 = Not Equal To 0?(x=w345) -> (x != 0?=w351:bool)
    n200 = Decrement(x=w353) -> (x-1=w354:u32)
    n201 = To Unsigned Byte Integer(number=w346) -> (unsigned 8bit integer=w349:u8)
    n202 = Increment(x=w353) -> (x+1=w352:u32)
    n203 = call <vilib>:"niFPGA Boolean Crossing.vi"("input"=w348, "direction"=w349) -> ("crossing"=w358:bool)  [unwired: 7 in]
    n204 = Select(t=w352, s=w351, f=w354) -> (s? t:f=w350:u32)
    n205 = Select(t=w350, s=w358, f=w353) -> (s? t:f=w357:u32)
    n206 = Select(t=u32 0, s=w344, f=w357) -> (s? t:f=w356:u32)
    "Count 2" <- w356
  }
  n207 = timed-loop "Timed Loop" {
    timing: w5 -> [_]
    timing-out: [_] -> w4
    shift-right: [w373] -> _
    shift-left: w1 -> [w370]
    stop <- FALSE stop-if-true
    # "3."
    # "4."
    # "2."
    # "1."
    # "Counter in a Single Cycle Timed Loop"
    n208 = xnode "FPGA I/O Node"() -> ("Mod5/DI4"=w365:bool)  [unwired: 1 in, 1 out]
    n209 = local read "Count Direction"() -> (w362:enum16{"Count Down", "Count Up"})
    n210 = local read "Edge"() -> (w363:enum8{"Either", "Rising Edge", "Falling Edge"})
    n211 = local read "Reset"() -> (w361:bool)
    n212 = Not Equal To 0?(x=w362) -> (x != 0?=w368:bool)
    n213 = Decrement(x=w370) -> (x-1=w371:u32)
    n214 = To Unsigned Byte Integer(number=w363) -> (unsigned 8bit integer=w366:u8)
    n215 = Increment(x=w370) -> (x+1=w369:u32)
    n216 = call <vilib>:"niFPGA Boolean Crossing.vi"("input"=w365, "direction"=w366) -> ("crossing"=w375:bool)  [unwired: 7 in]
    n217 = Select(t=w369, s=w368, f=w371) -> (s? t:f=w367:u32)
    n218 = Select(t=w367, s=w375, f=w370) -> (s? t:f=w374:u32)
    n219 = Select(t=u32 0, s=w361, f=w374) -> (s? t:f=w373:u32)
    "Count 5" <- w373
  }
  n220 = node-c288(w10) -> ()
  n221 = node-c288(w4) -> ()
  n222 = node-c288() -> (w9:T4)  [unwired: 1 in]
  n223 = node-c288() -> (w3:T4)  [unwired: 1 in]
  n224 = timed-loop "Timed Loop" {
    timing: w9 -> [_]
    timing-out: [_] -> w8
    shift-right: [w390] -> _
    shift-left: w1 -> [w387]
    stop <- FALSE stop-if-true
    # "3."
    # "4."
    # "2."
    # "1."
    # "Counter in a Single Cycle Timed Loop"
    n225 = xnode "FPGA I/O Node"() -> ("Mod5/DI2"=w382:bool)  [unwired: 1 in, 1 out]
    n226 = local read "Reset"() -> (w378:bool)
    n227 = local read "Count Direction"() -> (w380:enum16{"Count Down", "Count Up"})
    n228 = local read "Edge"() -> (w379:enum8{"Either", "Rising Edge", "Falling Edge"})
    n229 = Not Equal To 0?(x=w380) -> (x != 0?=w385:bool)
    n230 = Decrement(x=w387) -> (x-1=w388:u32)
    n231 = To Unsigned Byte Integer(number=w379) -> (unsigned 8bit integer=w383:u8)
    n232 = Increment(x=w387) -> (x+1=w386:u32)
    n233 = call <vilib>:"niFPGA Boolean Crossing.vi"("input"=w382, "direction"=w383) -> ("crossing"=w392:bool)  [unwired: 7 in]
    n234 = Select(t=w386, s=w385, f=w388) -> (s? t:f=w384:u32)
    n235 = Select(t=w384, s=w392, f=w387) -> (s? t:f=w391:u32)
    n236 = Select(t=u32 0, s=w378, f=w391) -> (s? t:f=w390:u32)
    "Count 3" <- w390
  }
  n237 = timed-loop "Timed Loop" {
    timing: w3 -> [_]
    timing-out: [_] -> w2
    shift-right: [w407] -> _
    shift-left: w1 -> [w404]
    stop <- FALSE stop-if-true
    # "3."
    # "4."
    # "2."
    # "1."
    # "Counter in a Single Cycle Timed Loop"
    n238 = xnode "FPGA I/O Node"() -> ("Mod5/DI3"=w399:bool)  [unwired: 1 in, 1 out]
    n239 = local read "Count Direction"() -> (w396:enum16{"Count Down", "Count Up"})
    n240 = local read "Reset"() -> (w395:bool)
    n241 = local read "Edge"() -> (w397:enum8{"Either", "Rising Edge", "Falling Edge"})
    n242 = Not Equal To 0?(x=w396) -> (x != 0?=w402:bool)
    n243 = Decrement(x=w404) -> (x-1=w405:u32)
    n244 = To Unsigned Byte Integer(number=w397) -> (unsigned 8bit integer=w400:u8)
    n245 = Increment(x=w404) -> (x+1=w403:u32)
    n246 = call <vilib>:"niFPGA Boolean Crossing.vi"("input"=w399, "direction"=w400) -> ("crossing"=w409:bool)  [unwired: 7 in]
    n247 = Select(t=w403, s=w402, f=w405) -> (s? t:f=w401:u32)
    n248 = Select(t=w401, s=w409, f=w404) -> (s? t:f=w408:u32)
    n249 = Select(t=u32 0, s=w395, f=w408) -> (s? t:f=w407:u32)
    "Count 4" <- w407
  }
  n250 = node-c288(w8) -> ()
  n251 = node-c288(w2) -> ()
